vi "QSPARK_setBatchPulseNumber.vi"(8 "Number of Pulses":i32, 11 "client handle":T1) -> (3 "client handle out":T1)   [LabVIEW 2024]
uses:
  <vilib>/httpClient/ClientHandle.ctl
  <vilib>/httpClient/LabVIEWHTTPClient.lvlib
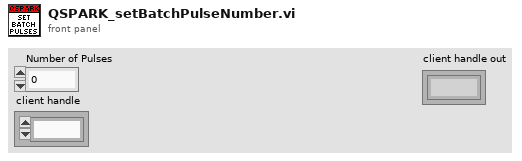
[diagram p1: front panel]
types:
  T1 = typedef "LabVIEWHTTPClient.lvlib/ClientHandle.ctl" = refnum<k1>
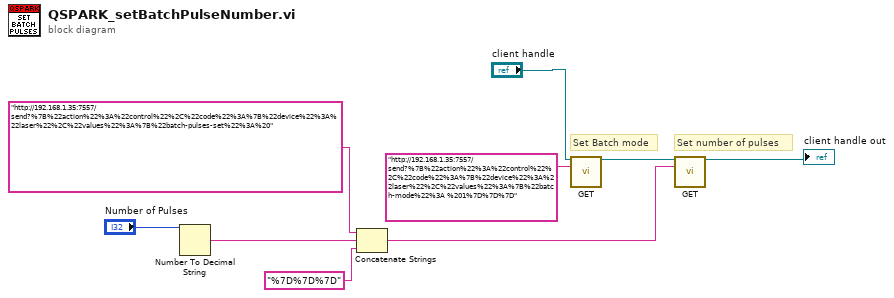
[diagram p0: block diagram]
diagram:
  # "Set Batch mode"
  # "Set number of pulses"
  n1 = Number To Decimal String(number="Number of Pulses") -> (decimal integer string=w3:string)  [unwired: 1 in]
  n2 = Concatenate Strings("http://192.168.1.35:7557/send?%7B%22action%22%3A%22control%22%2C%22code%22%3A%7B%22device%22%3A%22laser%22%2C%22values%22%3A%7B%22batch-pulses-set%22%3A%20" ("string"), w3, "%7D%7D%7D" ("string")) -> (w5:string)
  n3 = call <vilib>:"GET.vi"("client handle"="client handle", "url"="http://192.168.1.35:7557/send?%7B%22action%22%3A%22control%22%2C%22code%22%3A%7B%22device%22%3A%22laser%22%2C%22values%22%3A%7B%22batch-mode%22%3A %201%7D%7D%7D") -> ("client handle out"=w7:T1)  [unwired: 10 in, 3 out]
  n4 = call <vilib>:"GET.vi"("client handle"=w7, "url"=w5) -> ("client handle out"=→"client handle out":T1)  [unwired: 10 in, 3 out]
